vi "Configure Sweep Mode.vi"(8 "error in (no error)":errorcluster, 9 "Sweep Speed (1: Fast)":i32(ring)=1 items=["Normal", "Fast"], 10 "Sweep Mode (0: Sweep)":i32(ring) items=["Sweep", "FFT", "Auto"], 11 "VISA resource name":refnum<visa-resource-name>) -> (0 "error out":errorcluster, 3 "VISA resource name out":refnum<visa-resource-name>)   [LabVIEW 2022 SP3, in "Agilent N934X Series.lvlib"]
doc: "Configures the sweeping mode of the spectrum analyzer."
uses:
  <instrlib>/Agilent N934X Series/Agilent N934X Series.lvlib
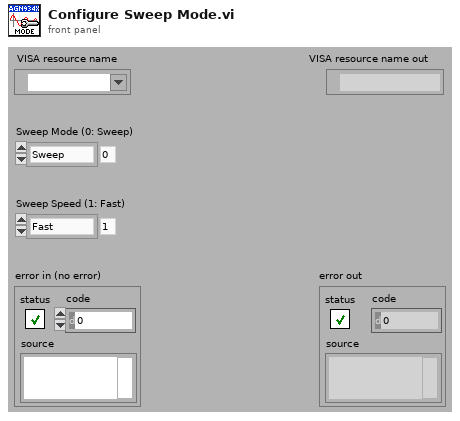
[diagram p1: front panel]
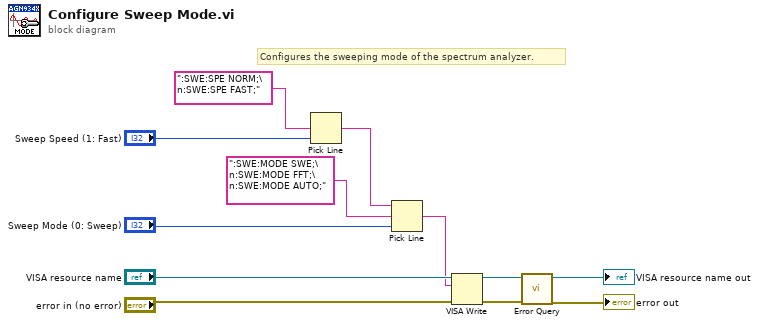
[diagram p0: block diagram]
diagram:
  # "Configures the sweeping mode of the spectrum analyzer."
  n1 = Pick Line(multi-line string=":SWE:SPE NORM;\n:SWE:SPE FAST;", line index="Sweep Speed (1: Fast)") -> (output string=w3:string)  [unwired: 1 in]
  n2 = Pick Line(string ("")=w3, multi-line string=":SWE:MODE SWE;\n:SWE:MODE FFT;\n:SWE:MODE AUTO;", line index="Sweep Mode (0: Sweep)") -> (output string=w1:string)
  n3 = VISA Write(VISA resource name="VISA resource name", write buffer=w1, error in (no error)="error in (no error)") -> (VISA resource name out=w8:refnum<visa-resource-name>, error out=w7:errorcluster)  [unwired: 1 out]
  n4 = call <instrlib>:"Error Query.vi"("error in (no error)"=w7, "VISA resource name"=w8) -> ("error out"=→"error out":errorcluster, "VISA resource name out"=→"VISA resource name out":refnum<visa-resource-name>)  [unwired: 6 in, 2 out]
